vi "Day 17 Testing Custom Boolean Gates Part 2.vi"() -> ()   [LabVIEW 2026]
panel:
  out "Array Y":bool[][][](array[boolean])
  out "XNOR Grid":bool[][](array[boolean])
  out "XOR Grid":bool[][](array[boolean])
  out "NOR Grid":bool[][](array[boolean])
  out "NAND Grid":bool[][](array[boolean])
  out "OUTPUT Y":bool
  in  "INPUT A  2":bool
  in  "INPUT B  2":bool
  out "OUTPUT":bool
  in  "INPUT A":bool
  in  "INPUT B":bool
  out "Output Y":bool
  in  "Input B 2":bool
  in  "Input A 2":bool
  out "Output":bool
  in  "Input B":bool
  in  "Input A":bool
  # "CUSTOM NAND GATE"
  # "CUSTOM NOR GATE"
  # "CUSTOM XOR GATE"
  # "CUSTOM XNOR GATE"
  # "CUSTOM NAND, NOR, XOR, NXOR  GATES VERIFICATION AGAINST  NATIVE TRUTH TABLE"
  # "y = ab + b ¯ c + c¯a¯"
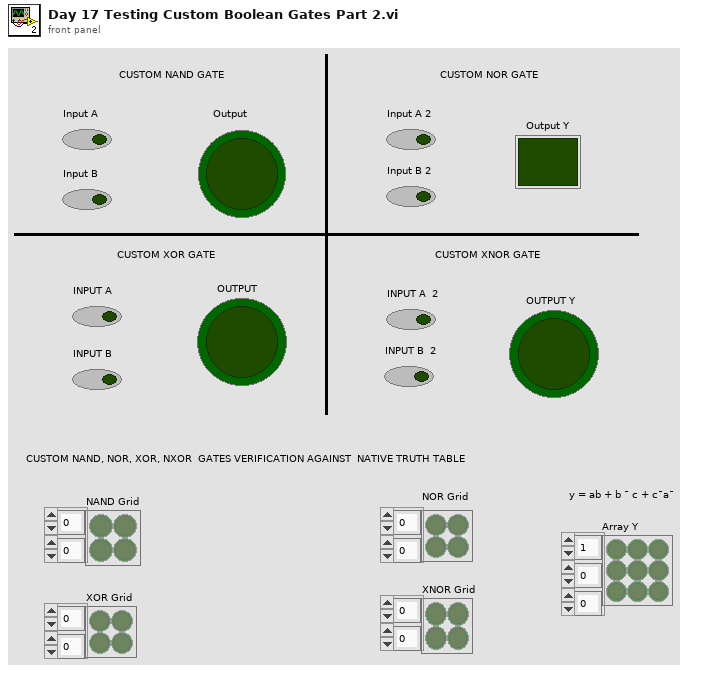
[diagram p1: front panel]
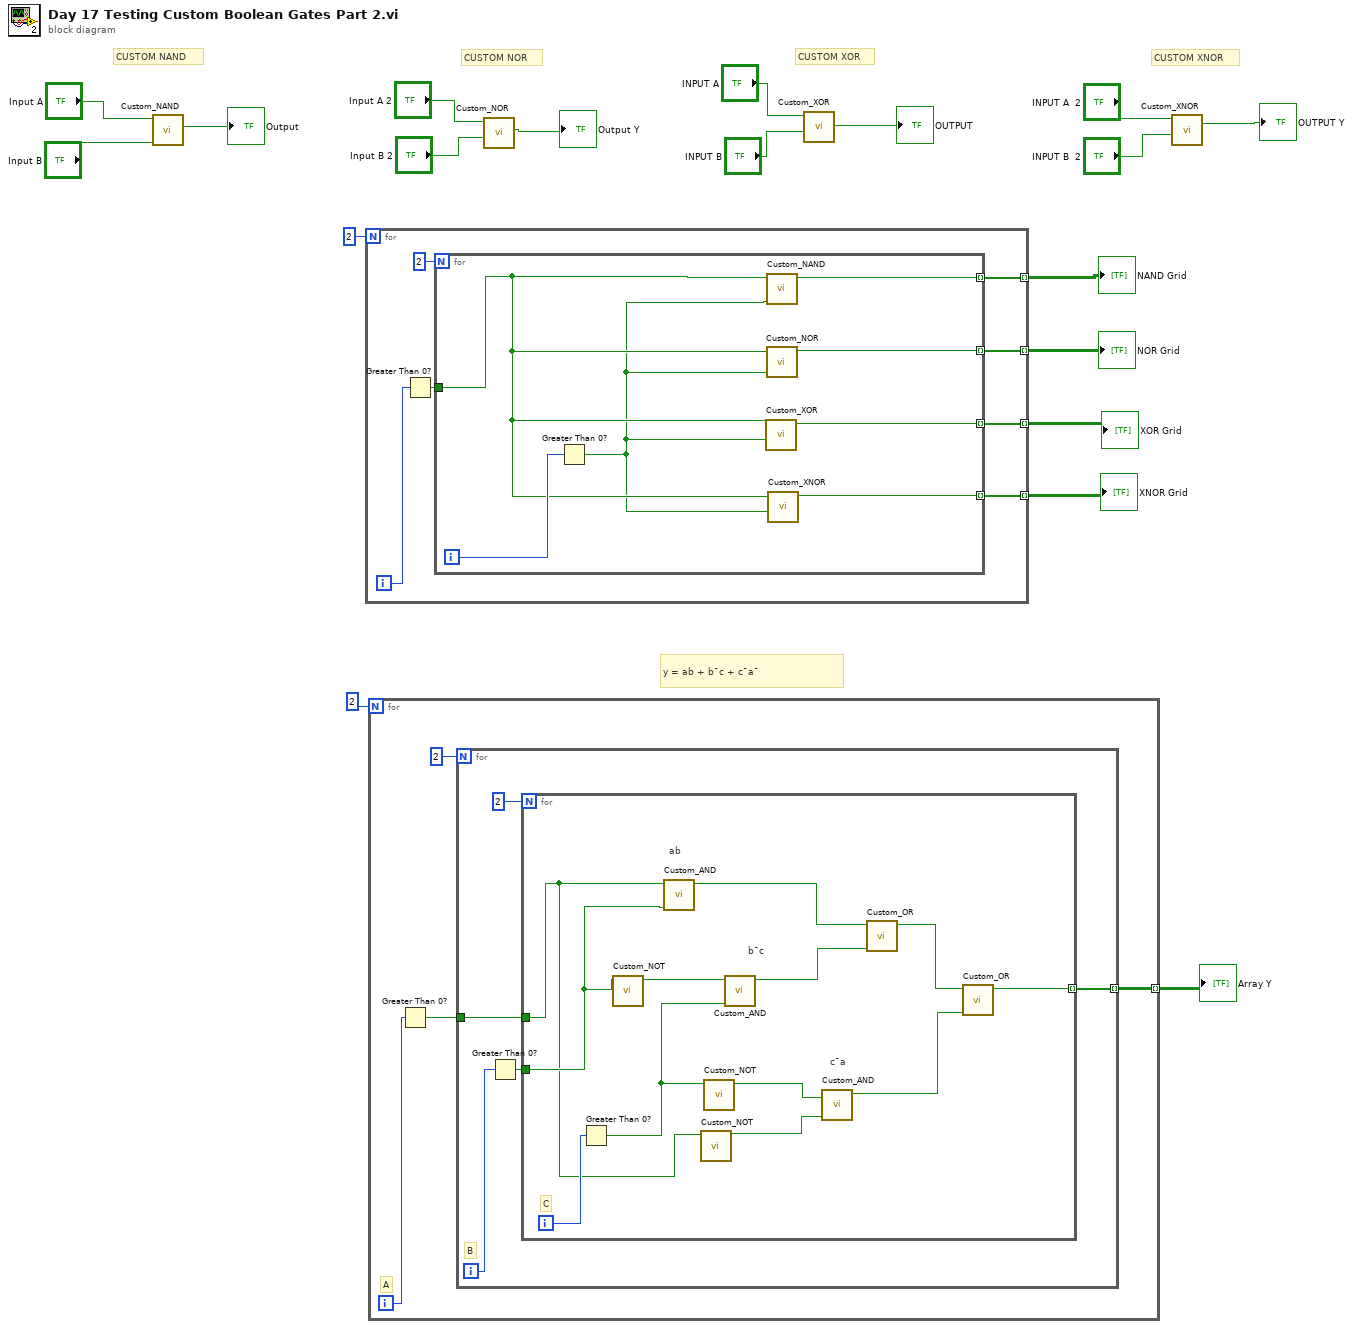
[diagram p0: block diagram]
diagram:
  # "y = ab + b¯c + c¯a¯"
  # "CUSTOM XNOR"
  # "CUSTOM XOR"
  # "CUSTOM NOR"
  # "CUSTOM NAND"
  n1 = call "Custom_NAND.vi"("Input B"="Input B", "Input A"="Input A") -> ("Output"=→"Output":bool)  [unwired: 9 in]
  n2 = for {
    N: 2 -> [_]
    tunnel: [w23] -> w8 mode=indexing
    tunnel: [w22] -> w7 mode=indexing
    tunnel: [w21] -> w6 mode=indexing
    tunnel: [w20] -> w5 mode=indexing
    i -> [w26]
    n3 = Greater Than 0?(x=w26) -> (x > 0?=w24:bool)
    n4 = for {
      N: 2 -> [_]
      tunnel: w24 -> [w32]
      tunnel: [w30] -> w23 mode=indexing
      tunnel: [w29] -> w22 mode=indexing
      tunnel: [w28] -> w21 mode=indexing
      tunnel: [w27] -> w20 mode=indexing
      i -> [w33]
      n5 = Greater Than 0?(x=w33) -> (x > 0?=w31:bool)
      n6 = call "Custom_XOR.vi"("INPUT B"=w31, "INPUT A"=w32) -> ("Boolean 3"=w28:bool)  [unwired: 9 in]
      n7 = call "Custom_NAND.vi"("Input B"=w31, "Input A"=w32) -> ("Output"=w30:bool)  [unwired: 9 in]
      n8 = call "Custom_NOR.vi"("Input B"=w31, "Input A"=w32) -> ("Output Y"=w29:bool)  [unwired: 9 in]
      n9 = call "Custom_XNOR.vi"("INPUT B"=w31, "INPUT A"=w32) -> ("Boolean 3"=w27:bool)  [unwired: 9 in]
    }
  }
  "NAND Grid" <- w8
  "NOR Grid" <- w7
  "XOR Grid" <- w6
  "XNOR Grid" <- w5
  n10 = for {
    N: 2 -> [_]
    tunnel: [w34] -> w1 mode=indexing
    i -> [w36]
    # "A"
    n11 = Greater Than 0?(x=w36) -> (x > 0?=w35:bool)
    n12 = for {
      N: 2 -> [_]
      tunnel: w35 -> [w40]
      tunnel: [w38] -> w34 mode=indexing
      i -> [w41]
      # "B"
      n13 = Greater Than 0?(x=w41) -> (x > 0?=w39:bool)
      n14 = for {
        N: 2 -> [_]
        tunnel: w40 -> [w50]
        tunnel: w39 -> [w53]
        tunnel: [w43] -> w38 mode=indexing
        i -> [w54]
        # "c¯a"
        # "b¯c"
        # "ab"
        # "C"
        n15 = Greater Than 0?(x=w54) -> (x > 0?=w51:bool)
        n16 = call "Custom_NOT.vi"("Input"=w53) -> ("Output"=w52:bool)  [unwired: 10 in]
        n17 = call "Custom_AND.vi"("Input B"=w53, "Input A"=w50) -> ("Output Y"=w47:bool)  [unwired: 9 in]
        n18 = call "Custom_NOT.vi"("Input"=w50) -> ("Output"=w48:bool)  [unwired: 10 in]
        n19 = call "Custom_NOT.vi"("Input"=w51) -> ("Output"=w49:bool)  [unwired: 10 in]
        n20 = call "Custom_AND.vi"("Input B"=w51, "Input A"=w52) -> ("Output Y"=w46:bool)  [unwired: 9 in]
        n21 = call "Custom_AND.vi"("Input B"=w48, "Input A"=w49) -> ("Output Y"=w44:bool)  [unwired: 9 in]
        n22 = call "Custom_OR.vi"("Input B"=w46, "Input A"=w47) -> ("Output Y"=w45:bool)  [unwired: 9 in]
        n23 = call "Custom_OR.vi"("Input B"=w44, "Input A"=w45) -> ("Output Y"=w43:bool)  [unwired: 9 in]
      }
    }
  }
  "Array Y" <- w1
  n24 = call "Custom_NOR.vi"("Input B"="Input B 2", "Input A"="Input A 2") -> ("Output Y"=→"Output Y":bool)  [unwired: 9 in]
  n25 = call "Custom_XOR.vi"("INPUT B"="INPUT B", "INPUT A"="INPUT A") -> ("Boolean 3"=→"OUTPUT":bool)  [unwired: 9 in]
  n26 = call "Custom_XNOR.vi"("INPUT B"="INPUT B  2", "INPUT A"="INPUT A  2") -> ("Boolean 3"=→"OUTPUT Y":bool)  [unwired: 9 in]
